vi "Make Sure Front Panel is open.vi"(0 "path":path) -> ()   [LabVIEW 2018]
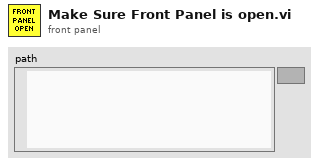
[diagram p1: front panel]
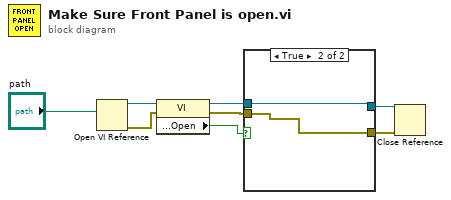
[diagram p0: block diagram]
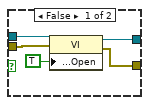
[diagram p2: hidden frame]
diagram:
  n1 = Open VI Reference(vi path="path") -> (vi reference=w2:refnum<vi>, error out=w6:errorcluster)  [unwired: 1 in, 4 out]
  n2 = property class="VI"(reference=w2, error in=w6) -> (reference out=w4:refnum<vi>, error out=w5:errorcluster, "Front Panel Window:Open"=w3:bool)
  n3 = case shown="True" w3 {
    tunnel: w4 -> [w13 w15]
    tunnel: w5 -> [w12 w14]
    tunnel: [w10 w15] -> w7
    tunnel: [w9 w14] -> w8
    frame False {
      n4 = property class="VI"(reference=w13, error in=w12, "Front Panel Window:Open"=TRUE) -> (reference out=w10:refnum<vi>, error out=w9:errorcluster)
    }
    frame True {
    }
  }
  n5 = Close Reference(reference=w7, error in (no error)=w8) -> ()  [unwired: 1 out]
